vi "tempcondqheat.vi"(1 "temp address":string) -> (0 "heater power":dbl format="%.2f")   [LabVIEW 2013]
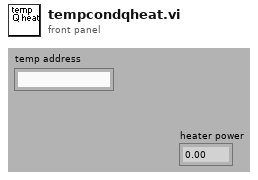
[diagram p1: front panel]
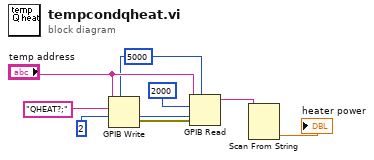
[diagram p0: block diagram]
diagram:
  w4 = 2
  w6 = 5000
  n1 = GPIB Write(0:"temp address", 1:"QHEAT?;", 2:w4, 4:w6) -> (6:w8:errorcluster)  [unwired: 1 in, 1 out]
  n2 = GPIB Read(0:"temp address", 1:2000, 2:w4, 3:w8, 4:w6) -> (5:w3:string)  [unwired: 2 out]
  n3 = Scan From String(input string=w3) -> (output 1=→"heater power":dbl)  [unwired: 4 in, 3 out]
